vi "tcp_disconnect.vi"(7 "button_tcp_disconnect":bool, 8 "error in":errorcluster, 9 "tcp_connected_in":bool, 11 "connection_id_in":refnum<k5>) -> (0 "error out":errorcluster, 1 "tcp_connected_out":bool, 3 "connection_id_out":refnum<k5>)   [LabVIEW 2025]
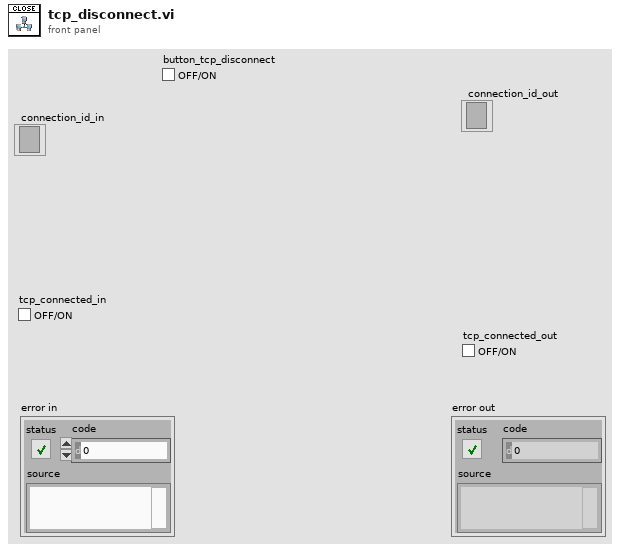
[diagram p1: front panel]
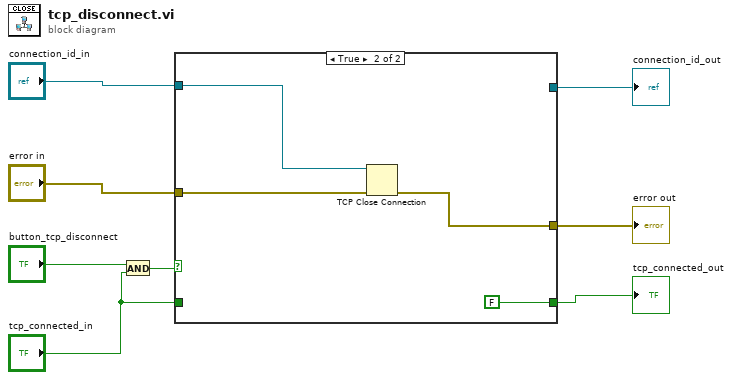
[diagram p0: block diagram]
diagram:
  n1 = And(x="button_tcp_disconnect", y="tcp_connected_in") -> (x .and. y?=w8:bool)
  n2 = case shown="True" w8 {
    tunnel: [w9 w14] -> w6
    tunnel: [w11 FALSE ("tcp_connected_in")] -> w5
    tunnel: "tcp_connected_in" -> [w11 _]
    tunnel: [w10 _] -> w4
    tunnel: "connection_id_in" -> [w10 w15]
    tunnel: "error in" -> [w9 w12]
    frame False {
    }
    frame True {
      n3 = TCP Close Connection(connection ID=w15, error in (no error)=w12) -> (error out=w14:errorcluster)  [unwired: 1 in, 1 out]
    }
  }
  "error out" <- w6
  "tcp_connected_out" <- w5
  "connection_id_out" <- w4
